vi "Do This.vi"(8 "error in (no error)":errorcluster, 10 "Status Events":refnum<class "Status Events.lvclass">, 11 "VIP Install in":refnum<class "VIP Install.lvclass">) -> (0 "error out":errorcluster, 3 "VIP Install out":refnum<class "VIP Install.lvclass">)   [LabVIEW 2014, in "VIP Install.lvclass"]
uses:
  VIP Install.lvclass
  Classes/Status Events/Status Events.lvclass
  VIP Install.lvclass/VIP Install.ctl
  <vilib>/Utility/error.llb/DialogType.ctl
  Classes/Job/Job.lvclass/Job.ctl
  <vilib>/JKI/VIPM API/VIPM API_vipm_api.lvlib
  Classes/Job/Job.lvclass
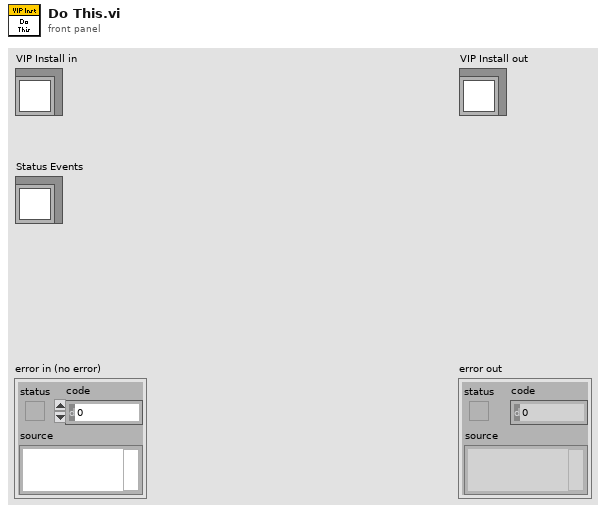
[diagram p1: front panel]
types:
  T1 = typedef "VIPM API_vipm_api.lvlib/Library Contents Cluster_vipm_api.ctl" = cluster{"Package Name":string, "Version":string, "Display Name":string, "Repository Name":string, "Company Name":string, "License Type":string, "Installed":bool, "Deprecated":bool, "Dependency or Conflict Problem":bool, "Downloaded":bool}
  T2 = typedef "DialogType.ctl" = u16
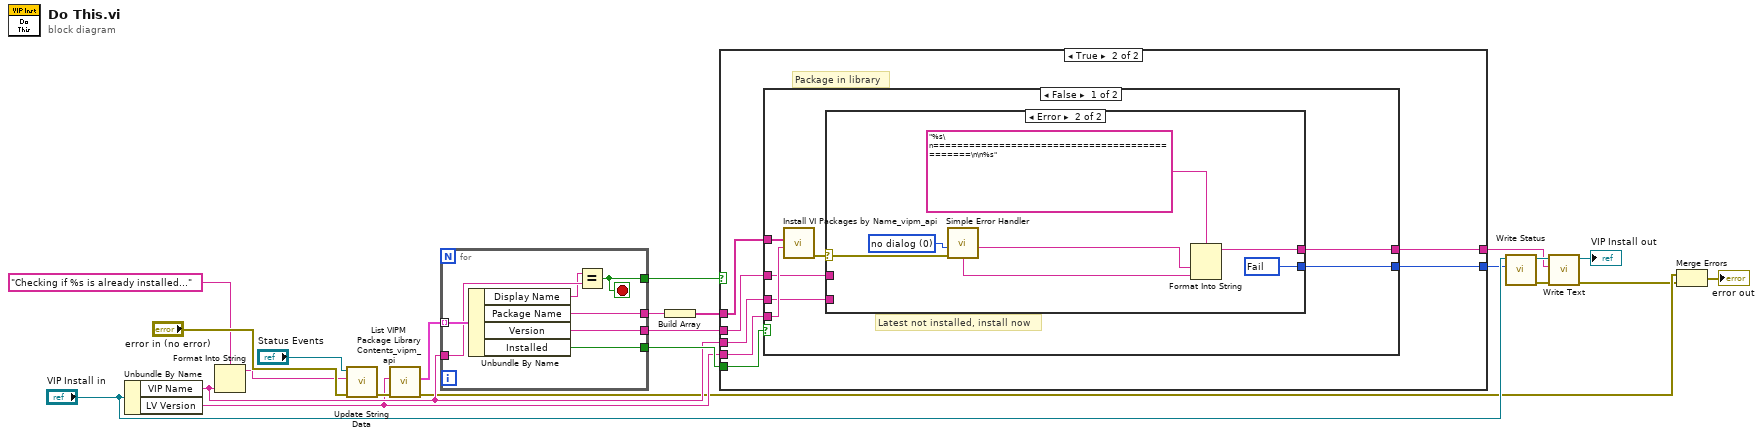
[diagram p0: block diagram]
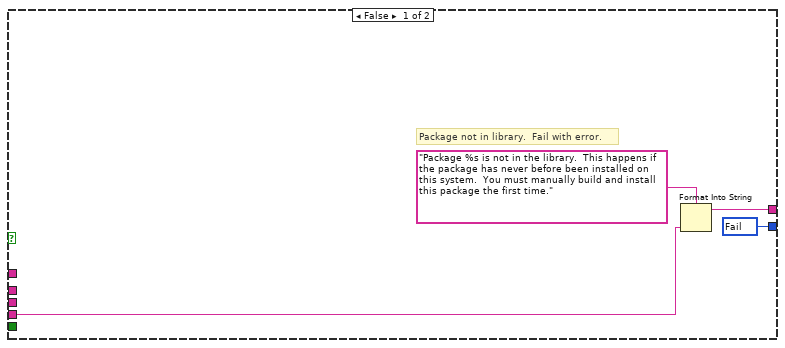
[diagram p2: hidden frame]
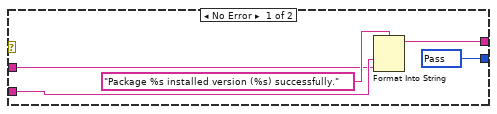
[diagram p3: hidden frame]
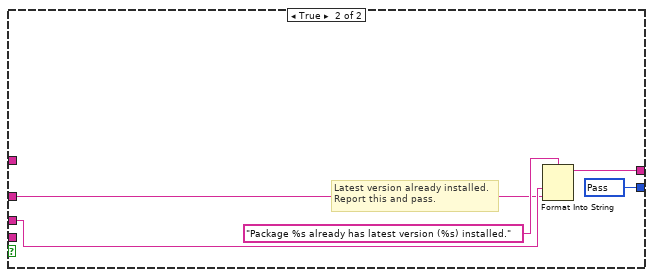
[diagram p4: hidden frame]
diagram:
  n1 = Unbundle By Name("VIP Install in") -> ("VIP Name"=w10:string, "LV Version"=w7:string)
  n2 = Format Into String(format string="Checking if %s is already installed...", w10) -> (resulting string=w19:string)  [unwired: 2 in, 1 out]
  n3 = call "Update String Data.vi"("error in (no error)"="error in (no error)", "String Data"=w19, "Status Updater in"="Status Events") -> ("error out"=w18:errorcluster)  [unwired: 7 in, 1 out]
  n4 = call <vilib>:"List VIPM Package Library Contents_vipm_api.vi"("error in (no error)"=w18, "LabVIEW Version"=w7) -> ("error out"=w4:errorcluster, "Library Contents []"=w17:T1[])  [unwired: 8 in]
  n5 = for {
    tunnel: w17 -> [w29] mode=indexing
    tunnel: w10 -> [w28]
    tunnel: [w27] -> w15
    tunnel: [w26] -> w9
    tunnel: [w25] -> w16
    tunnel: [w24] -> w1
    stop <- w25 stop-if-true
    n6 = Unbundle By Name(w29) -> ("Display Name"=w23:string, "Package Name"=w24:string, "Version"=w26:string, "Installed"=w27:bool)
    n7 = Equal?(x=w23, y=w28) -> (x = y?=w25:bool)
  }
  n8 = Build Array(w1) -> (w8:string[])
  n9 = case shown="True" w16 {
    tunnel: w15 -> [_ w40]
    tunnel: w10 -> [_ w39]
    tunnel: w9 -> [_ w38]
    tunnel: [w33 w37] -> w6
    tunnel: w8 -> [_ w36]
    tunnel: w7 -> [w30 w35]
    tunnel: [w31 w34] -> w5
    frame False {
      w33 = u16 500 items=["Abort"=503, "Fail"=500, "Pass"=200] ("Status")
      # "Package not in library.  Fail with error."
      n10 = Format Into String(format string="Package %s is not in the library.  This happens if the package has never before been installed on this system.  You must manually build and install this package the first time.", w30) -> (resulting string=w31:string)  [unwired: 2 in, 1 out]
    }
    frame True {
      # "Package in library"
      n11 = case shown="False" w40 {
        tunnel: w39 -> [w42 w63]
        tunnel: w38 -> [w41 w62]
        tunnel: [w44 w61] -> w37
        tunnel: w36 -> [w47 _]
        tunnel: w35 -> [w46 _]
        tunnel: [w43 w60] -> w34
        frame False {
          # "Latest not installed, install now"
          n12 = call <vilib>:"Install VI Packages by Name_vipm_api.vi"("LabVIEW Version"=w46, "Package Names to Install []"=w47) -> ("error out"=w45:errorcluster)  [unwired: 9 in]
          n13 = case shown="Error" w45 {
            selector: w45 -> [_ w53]
            tunnel: [w52 w59] -> w44
            tunnel: [w50 w54] -> w43
            tunnel: w42 -> [w49 _]
            tunnel: w41 -> [w48 _]
            frame No Error {
              w52 = u16 200 items=["Abort"=503, "Fail"=500, "Pass"=200] ("Status")
              n14 = Format Into String(format string="Package %s installed version (%s) successfully.", w49, w48) -> (resulting string=w50:string)  [unwired: 2 in, 1 out]
            }
            frame Error {
              w55 = T2 0 items=["no dialog", "OK message", "continue or stop message", "OK message + warnings", "continue/stop + warnings"] ("type of dialog (OK msg:1)")
              w59 = u16 500 items=["Abort"=503, "Fail"=500, "Pass"=200] ("Status")
              n15 = call <vilib>:"Simple Error Handler.vi"("type of dialog (OK msg:1)"=w55, "error in (no error)"=w53) -> ("source out"=w57:string, "message"=w58:string)  [unwired: 3 in, 3 out]
              n16 = Format Into String(format string="%s\n==============================================\n\n%s", w57, w58) -> (resulting string=w54:string)  [unwired: 2 in, 1 out]
            }
          }
        }
        frame True {
          w61 = u16 200 items=["Abort"=503, "Fail"=500, "Pass"=200] ("Status")
          # "Latest version already installed.\nReport this and pass."
          n17 = Format Into String(format string="Package %s already has latest version (%s) installed.", w63, w62) -> (resulting string=w60:string)  [unwired: 2 in, 1 out]
        }
      }
    }
  }
  n18 = call "Write Status.vi"("Status"=w6, "Job in"="VIP Install in") -> ("error out"=w12:errorcluster, "Job out"=w13:refnum<class "VIP Install.lvclass">)  [unwired: 8 in]
  n19 = call "Write Text.vi"("error in (no error)"=w12, "Text"=w5, "Job in"=w13) -> ("error out"=w3:errorcluster, "Job out"=→"VIP Install out":refnum<class "VIP Install.lvclass">)  [unwired: 7 in]
  n20 = Merge Errors(w4, w3) -> (→"error out":errorcluster)
